vi "uService GUI.vi"(8 "error in (no error)":errorcluster, 11 "uService Template in":refnum<class "Guardian Subpanel.lvclass">) -> (3 "uService Template out":refnum<class "Guardian Subpanel.lvclass">)   [LabVIEW 2026, in "TALOS.lvlib" / "Guardian Subpanel.lvlib" / "Guardian Subpanel.lvclass"]
uses:
  Guardian Subpanel.lvclass
  C:/LabVIEW Code/TALOS/talos/Father of all uServices/Father of all uServices/Father of all uServices.lvclass
  Ancestor/Ancestor/Ancestor.lvclass/Ancestor.ctl
  Support VIs/Substitute Error.vi
  Support VIs/Generate Error.vi
  FGV/Error Memory/Get Error Description.vi
  Support VIs/Get PC name.vi
  Ancestor/Ancestor/Read ID.vi
  Support VIs/Get Class Name.vi
  FGV/Error Memory/Error Memory Core.vi
  <vilib>/AdvancedString/Delimited String to 1D String Array.vi
  <vilib>/AdvancedString/Delimited String to 1D String Array (string).vi
  Support VIs/Circus Root Path.vi
  FGV/Error Memory/Error Crt Lvl checker.vi
  FGV/Error Memory/Error Memory Core.vi/40c8088d-b597-4017-91af-faa98e00292e.vi
  FGV/Error Memory/Error Memory Core.vi/d4a3ab98-063c-4e44-b43d-fbdcfe6c2be2.vi
  Father of all uServices/Father of all uServices/Father of all uServices.lvclass
  C:/LabVIEW Code/TALOS/builds/Actor Framework PPL/Actor Framework.lvlibp/1abvi3w/vi.lib/ActorFramework/Actor/Actor.lvclass
  builds/Actor Framework PPL/Actor Framework.lvlibp/1abvi3w/vi.lib/ActorFramework/Actor/Read Self Enqueuer.vi
  builds/Actor Framework PPL/Actor Framework.lvlibp/1abvi3w/vi.lib/ActorFramework/Stop Msg/Send Normal Stop.vi
  Support VIs/Global Memory.vi
  <vilib>/Utility/LVClass/Get LV Class Name.vi
  Support VIs/Is in Packed Library.vi
  Support VIs/TALOS Root path.vi
  Support VIs/Read CSV worksheet.vi
  Support VIs/Global Constants.vi
  <vilib>/Utility/error.llb/General Error Handler.vi
  Support VIs/Error Log.vi
  Ancestor/Ancestor/Ancestor.lvclass
  <vilib>/Comparison/Equal/Equal Functor/Equal Functor.lvclass
panel:
  in  "git branch name":string
  in  "Send I Exist":bool
  in  "Check Bearer":bool
  out "Bearer":string
  in  "Dismiss All Errors":bool
  in  "overwrite name":string
  in  "Enable Msg received":bool
  in  "Include critical PCs":bool
  in  "Update from GIT":bool
  in  "Reload INI files":bool
  in  "Reset ABORT":bool
  in  "Send Pat to all GDs":bool
  out "Message received":string
  in  "Stop online checks":bool
  in  "Start online checks":bool
  in  "uService":string
  in  "Stop uService":bool
  in  "Start uService":bool
  in  "Stop":bool
  out "uService ID":string
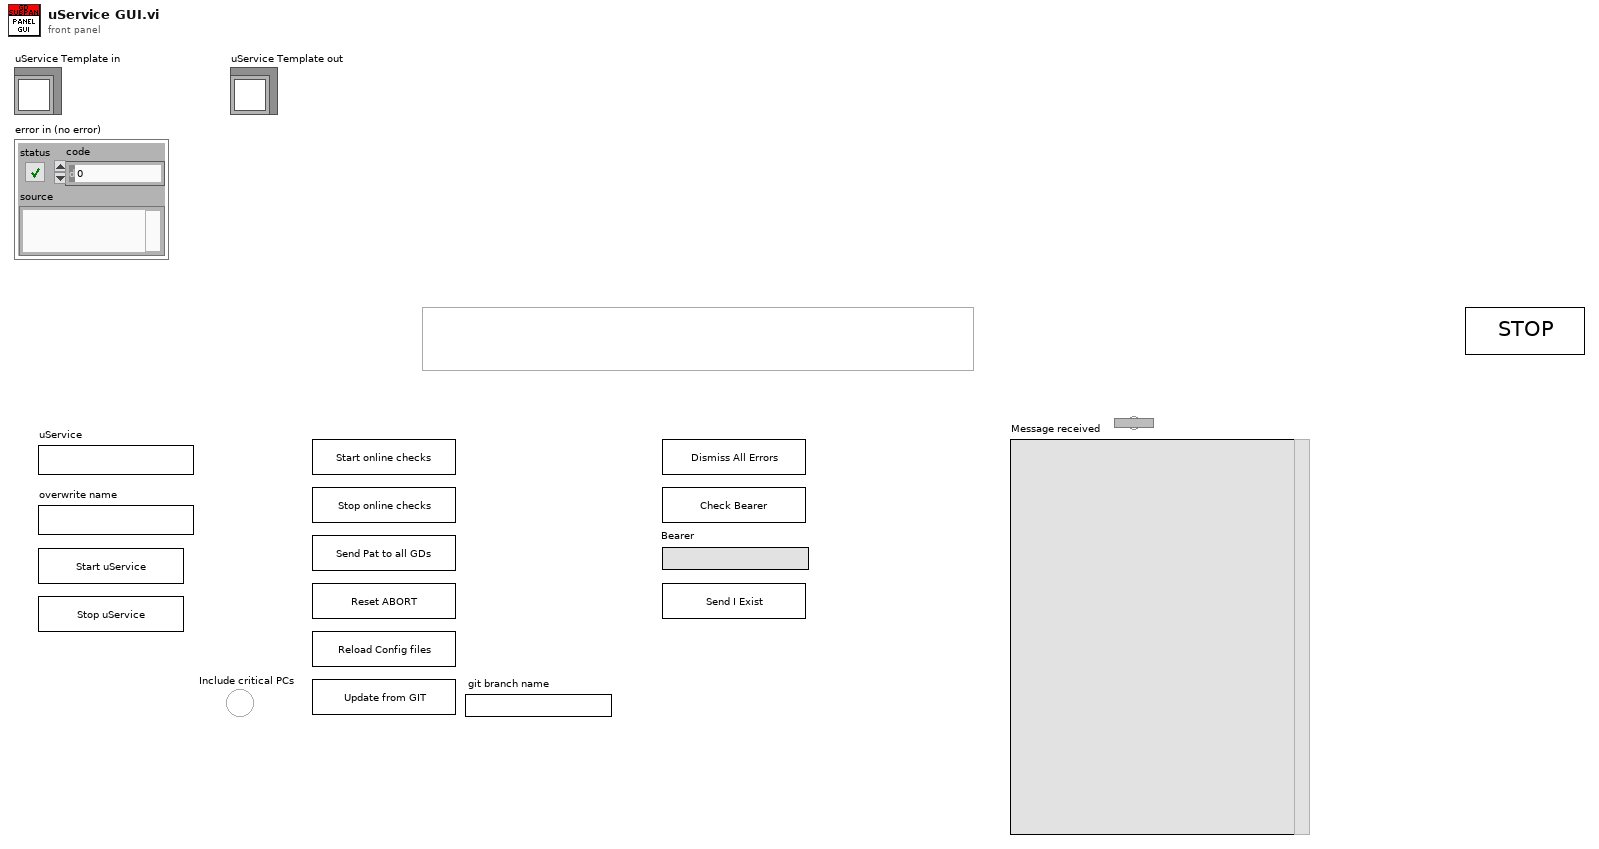
[diagram p1: front panel]
types:
  T1 = typedef "eventvkey.ctl" = enum16{"ASCII", "Enter", "Return", "Shift", "Ctrl", "Alt", "Cmd", "Opt", "Caps", "NumLock", "Clear", "Break", "Up", "Down", "Left", "Right", "Insert", "Delete", "Home", "End", "PageUp", "PageDown", "Escape", "Help", "Pause", "ScrollLock", "F1", "F2", "F3", "F4", "F5", "F6", "F7", "F8", "F9", "F10", "F11", "F12", "F13", "F14", "F15", "F16", "F17", "F18", "F19", "F20", "F21", "F22", "F23", "F24", "Play", "VolumeUp", "VolumeDown", "Mute", "Two Byte Char"}
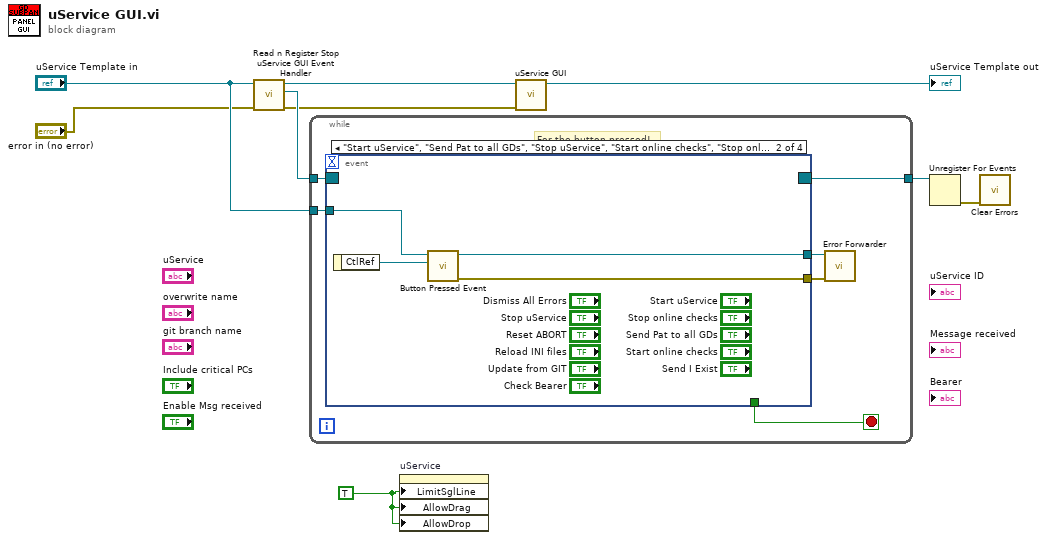
[diagram p0: block diagram]
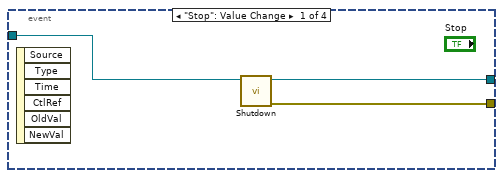
[diagram p2: hidden frame]
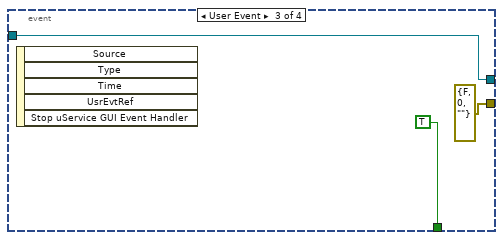
[diagram p3: hidden frame]
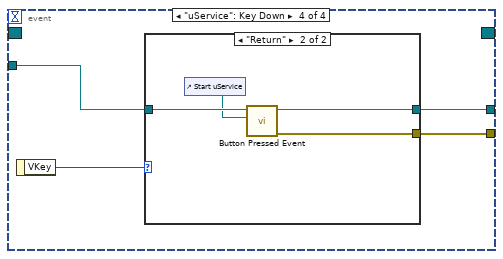
[diagram p4: hidden frame]
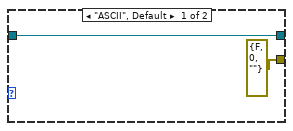
[diagram p5: hidden frame]
diagram:
  w6 = TRUE ("Limit To Single Line?")
  n1 = call-dynamic "Read n Register Stop uService GUI Event Handler .vi"("error in (no error)"="error in (no error)", "uService Template in"="uService Template in") -> ("error out"=w2:errorcluster, "Stop uService GUI Event Ref"=w7:refnum<event-registration>, "uService Template out"=w4:refnum<class "Guardian Subpanel.lvclass">)  [unwired: 7 in]
  n2 = while {
    tunnel: [w15] -> w8
    tunnel: "uService Template in" -> [w13]
    tunnel: w7 -> [w12]
    stop <- w14 stop-if-true
    # "For the button pressed!"
    n3 = event shown="[1] \"Start uService\", \"Send Pat to all GDs\", \"Stop uService\", \"Start online checks\", \"Stop online checks\", \"Reset ABORT\", \"Reload INI files\", \"Update from GIT\", \"Dismiss All Errors\", \"Check Bearer\", \"Send I Exist\": Value Change" {
      selector: w12 -> [_ _ _ _]
      dyn-events: [_ _ _ _] -> w15
      timeout: _ -> [_ _ _ _]
      tunnel: w13 -> [w18 w21 w24 w29]
      tunnel: [_ _ TRUE _] -> w14
      tunnel: [w17 w20 w24 w27] -> w11
      tunnel: [w16 w19 errorcluster {"status"=FALSE, "code"=0, "source"=""} ("error out") w26] -> w10
      event "Stop": Value Change {
        n4 = event-data() -> ()  [unwired: 1 in, 6 out]
        n5 = call "Shutdown.vi"("Father of all uServices in"=w18) -> ("error out"=w16:errorcluster, "Father of all uServices out"=w17:refnum<class "Guardian Subpanel.lvclass">)  [unwired: 9 in]
      }
      event "Start uService", "Send Pat to all GDs", "Stop uService", "Start online checks", "Stop online checks", "Reset ABORT", "Reload INI files", "Update from GIT", "Dismiss All Errors", "Check Bearer", "Send I Exist": Value Change {
        n6 = event-data() -> ("CtlRef"=w22:refnum<vi>)  [unwired: 1 in]
        n7 = call-dynamic "Button Pressed Event.vi"("CtlRef"=w22, "uService Template in"=w21) -> ("error out"=w19:errorcluster, "uService Template out"=w20:refnum<class "Guardian Subpanel.lvclass">)  [unwired: 8 in]
      }
      event User Event {
        n8 = event-data() -> ()  [unwired: 1 in, 5 out]
      }
      event "uService": Key Down {
        n9 = event-data() -> ("VKey"=w28:T1)  [unwired: 1 in]
        n10 = case shown="\"Return\"" w28 {
          tunnel: w29 -> [w31 w35]
          tunnel: [w31 w33] -> w27
          tunnel: [errorcluster {"status"=FALSE, "code"=0, "source"=""} ("error out") w32] -> w26
          frame "ASCII", Default {
          }
          frame "Return" {
            n11 = control-ref of="Start uService"() -> (w34:refnum<vi>)
            n12 = call-dynamic "Button Pressed Event.vi"("CtlRef"=w34, "uService Template in"=w35) -> ("error out"=w32:errorcluster, "uService Template out"=w33:refnum<class "Guardian Subpanel.lvclass">)  [unwired: 8 in]
          }
        }
      }
    }
    n13 = call "Error Forwarder.vi"("error in (no error)"=w10, "Father of all uServices in"=w11) -> ()  [unwired: 10 in]
  }
  n14 = property on="uService" class="Str"("LimitSglLine"=w6, "AllowDrag"=w6, "AllowDrop"=w6) -> ()  [unwired: 2 in, 2 out]
  n15 = call-parent "uService GUI.vi"("error in (no error)"=w2, "uService Template in"=w4) -> ("uService Template out"=→"uService Template out":refnum<class "Guardian Subpanel.lvclass">)  [unwired: 9 in]
  n16 = Unregister For Events(event registration refnum=w8) -> (error out=w1:errorcluster)  [unwired: 1 in]
  n17 = call <vilib>:"Clear Errors.vi"("error in (no error)"=w1) -> ()  [unwired: 5 in, 2 out]
